vi "Get UI Details.vi"(8 "error in":errorcluster, 11 "gRPC Server in":refnum<class "MeasurementPluginService.lvclass">) -> (0 "error out":errorcluster, 2 "user_interface_details":T1[](array[typedef]), 3 "gRPC Server out":refnum<class "MeasurementPluginService.lvclass">)   [LabVIEW 2020, in "MeasurementLink Measurement Server.lvlib" / "MeasurementPluginService.lvclass"]
uses:
  MeasurementPluginService.lvclass
  MeasurementLink Measurement Server Internal/RPC Messages/ni_measurementlink_measurement_v1_UserInterfaceDetails.ctl
  MeasurementPluginService.lvclass/MeasurementPluginService.ctl
  MeasurementLink Measurement Server Internal/MeasurementLink Measurement Server Internal.lvlib
  Helpers/TypeDefs/UI Information.ctl
  MeasurementLink Measurement Server.lvlib
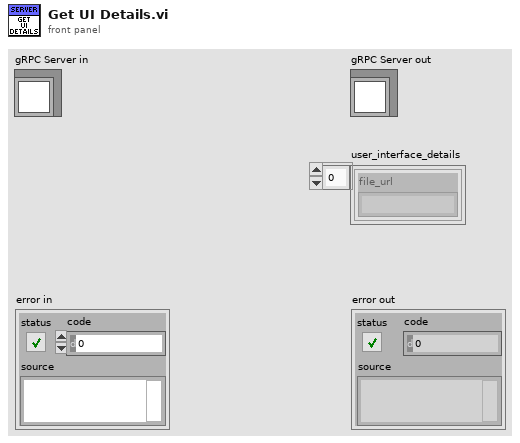
[diagram p1: front panel]
types:
  T1 = typedef "MeasurementLink Measurement Server Internal.lvlib/ni_measurementlink_measurement_v1_UserInterfaceDetails.ctl" = cluster{"file_url":string}
  T2 = typedef "MeasurementLink Measurement Server.lvlib/UI Information.ctl" = cluster{"File":string}
  T3 = typedef "MeasurementLink Measurement Server.lvlib/MeasurementPluginService.lvclass/Plugin Paths.ctl" = cluster{"Get Measurement Details VI Path":path, "Get Type Specializations VI Path":path, "Get UI Details VI Path":path, "Measurement Logic VI Path":path, "Measurement Configuration CTL Path":path, "Measurement Results CTL Path":path}
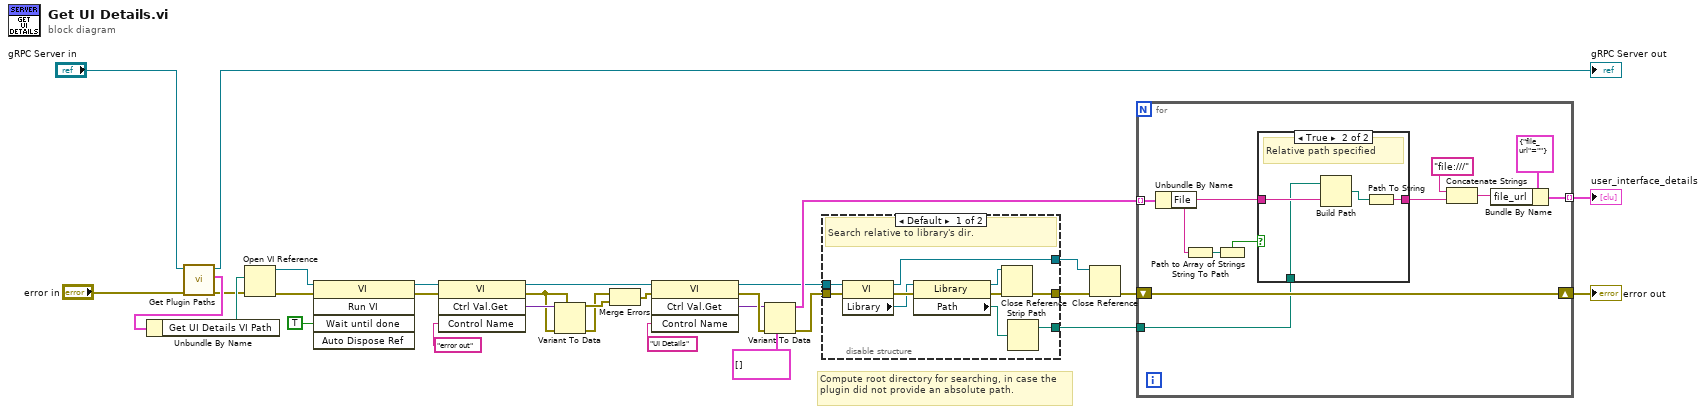
[diagram p0: block diagram]
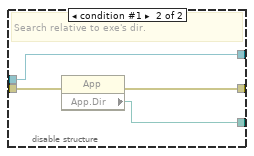
[diagram p2: hidden frame]
diagram:
  # "Compute root directory for searching, in case the plugin did not provide an absolute path."
  n1 = call-dynamic "Get Plugin Paths.vi"("error in (no error)"="error in", "MeasurementService in"="gRPC Server in") -> ("error out"=w25:errorcluster, "Plugin Paths"=w27:T3, "MeasurementService out"=→"gRPC Server out":refnum<class "MeasurementPluginService.lvclass">)  [unwired: 7 in]
  n2 = Unbundle By Name(w27) -> ("Get UI Details VI Path"=w26:path)
  n3 = Open VI Reference(vi path=w26, error in (no error)=w25) -> (vi reference=w8:refnum<vi>, error out=w9:errorcluster)  [unwired: 4 in]
  n4 = invoke class="VI" method="Run VI"(reference=w8, error in=w9, "Wait until done"=TRUE ("Wait Until Done")) -> (reference out=w15:refnum<vi>, error out=w14:errorcluster)  [unwired: 2 in, 3 out]
  n5 = invoke class="VI" method="Ctrl Val.Get"(reference=w15, error in=w14, "Control Name"="error out") -> (reference out=w11:refnum<vi>, error out=w20:errorcluster, "Get Control Value Variant"=w21:variant)  [unwired: 1 in, 1 out]
  n6 = Variant To Data(error in=w20, type=w20, Variant=w21) -> (data=w19:errorcluster, error out=w10:errorcluster)
  n7 = Merge Errors(w10, w19) -> (w13:errorcluster)
  n8 = invoke class="VI" method="Ctrl Val.Get"(reference=w11, error in=w13, "Control Name"="UI Details") -> (reference out=w6:refnum<vi>, error out=w18:errorcluster, "Get Control Value Variant"=w16:variant)  [unwired: 1 in, 1 out]
  n9 = Variant To Data(error in=w18, type=T2[] [], Variant=w16) -> (data=w12:T2[], error out=w7:errorcluster)
  n10 = disable-structure shown="Default" {
    disable-tunnel: w7 -> [w41 w44]
    disable-tunnel: [w35 w43] -> w4
    disable-tunnel: w6 -> [w40 w45]
    disable-tunnel: [w39 w45] -> w5
    disable-tunnel: [w32 w42] -> w1
    frame condition #0 (active) {
      # "Search relative to library's dir."
      n11 = property class="VI"(reference=w40, error in=w41) -> (reference out=w39:refnum<vi>, error out=w38:errorcluster, "Library"=w37:refnum<vi>)
      n12 = property class="Library"(reference=w37, error in=w38) -> (reference out=w34:refnum<vi>, error out=w36:errorcluster, "Path"=w33:path)
      n13 = Close Reference(reference=w34, error in (no error)=w36) -> (error out=w35:errorcluster)
      n14 = Strip Path(path=w33) -> (stripped path=w32:path)  [unwired: 1 out]
    }
    frame condition #1 {
      # "Search relative to exe's dir."
      n15 = property class="App"(error in=w44) -> (error out=w43:errorcluster, "App.Dir"=w42:path)  [unwired: 1 in, 1 out]
    }
  }
  n16 = Close Reference(reference=w5, error in (no error)=w4) -> (error out=w3:errorcluster)
  n17 = for {
    tunnel: w12 -> [w52] mode=indexing
    tunnel: [w53] -> w28 mode=indexing
    shift-right: [w49] -> w2
    shift-left: w3 -> [w49]
    tunnel: w1 -> [w48]
    n18 = Unbundle By Name(w52) -> ("File"=w47:string)
    n19 = String To Path(string=w47) -> (path=w51:path)
    n20 = Path to Array of Strings(0:w51) -> (1:w50:bool)  [unwired: 1 out]
    n21 = case shown="True" w50 {
      tunnel: w48 -> [_ w60]
      tunnel: w47 -> [w57 w61]
      tunnel: [w57 w58] -> w46
      frame False {
        # "absolute path specified"
      }
      frame True {
        # "Relative path specified"
        n22 = Build Path(base path=w60, name or relative path=w61) -> (appended path=w59:path)
        n23 = Path To String(path=w59) -> (string=w58:string)
      }
    }
    n24 = Concatenate Strings("file:///" ("string"), w46) -> (w55:string)
    n25 = Bundle By Name(cluster=T1 {"file_url"=""} ("UserInterfaceDetails"), "file_url"=w55) -> (w53:T1)
  }
  "error out" <- w2
  "user_interface_details" <- w28
